vi "Copy from excel - paste to LV table.vi"() -> ()   [LabVIEW 2010]
panel:
  in  "stop":bool
  in  "Paste":bool
  in  "Table Control":string[][](table)
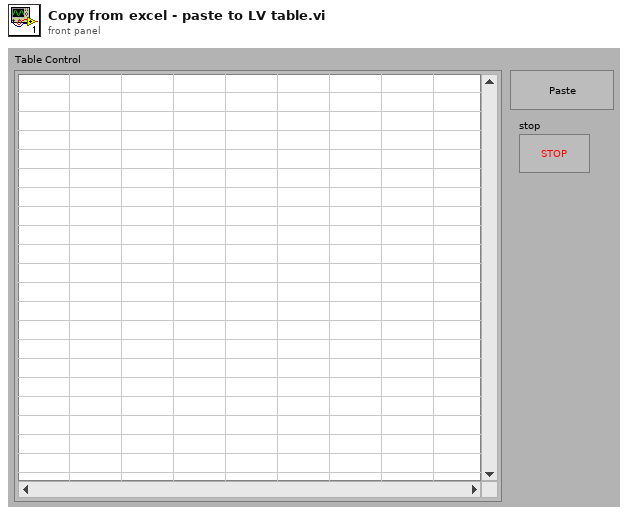
[diagram p1: front panel]
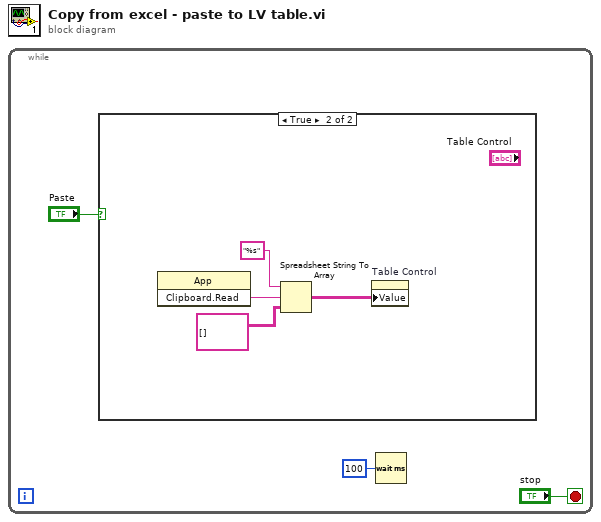
[diagram p0: block diagram]
diagram:
  n1 = while {
    stop <- "stop" stop-if-true
    n2 = case shown="True" "Paste" {
      frame False {
      }
      frame True {
        n3 = invoke class="App" method="Clipboard.Read"() -> ("Read Clipbrd"=w7:string)  [unwired: 3 in, 2 out]
        n4 = Spreadsheet String To Array(format string="%s", spreadsheet string=w7, array type (2D Dbl)=string[][] []) -> (array=w5:string[][])  [unwired: 1 in]
        n5 = property on="Table Control" class="Tbl (strict)"("Value"=w5) -> ()  [unwired: 2 in, 2 out]
      }
    }
    n6 = Wait (ms)(milliseconds to wait=u32 100) -> ()  [unwired: 1 out]
  }
